vi "GetText.vi"(8 "error in":errorcluster, 11 "Submodule EOL":refnum<class "Submodule EOL.lvclass">) -> (0 "error out":errorcluster, 1 "additional text":string, 2 "text":string, 3 "Submodule EOL out":refnum<class "Submodule EOL.lvclass">, 4 "glyph":string)   [LabVIEW 2025, in "Submodule EOL.lvlib" / "Submodule EOL.lvclass"]
doc: "Returns the text representation of the node used for the tree control.Copyright 2017 National Instruments Corporation\n\nLicensed under the Apache License, Version 2.0 (the \"License\"); you may not use this file except in compliance with the License. You may obtain a copy of the License at http://www.apache.org/licenses/LICENSE-2.0\nUnless required by applicable law or agreed to in writing, software distributed under the License is distributed on an \"AS IS\" BASIS, WITHOUT WARRANTIES OR CONDITIONS OF ANY KIND, either express or implied. See the License for the specific language governing permissions and limitations under the License."
uses:
  Submodule EOL.lvclass
  Submodule EOL.lvclass/Submodule EOL.ctl
  Submodule EOL configuration/Submodule EOL configuration.lvclass/Submodule EOL configuration.ctl
  Submodule EOL configuration/Read Submodule EOL.vi
  Submodule EOL configuration/Submodule EOL configuration.lvclass
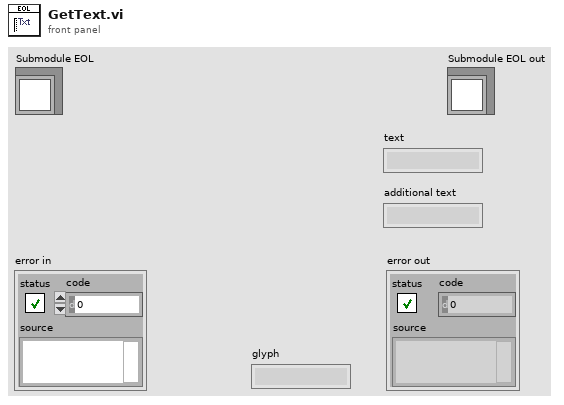
[diagram p1: front panel]
types:
  T1 = typedef "Submodule EOL.lvlib/Submodule EOL configuration.lvclass/Submodule EOL.ctl" = cluster{"PLC Folder Names":string[][], "Timeout Connect OPC":dbl, "Connect OPC Trial":u32, "PLC URL":string, "Digitial IO":string, "HiPOT":string, "ACIR with Switch":string, "DMM with Switch":string, "Ignition Folder Names":string[][], "Ignition URL":string, "Test Name":string}
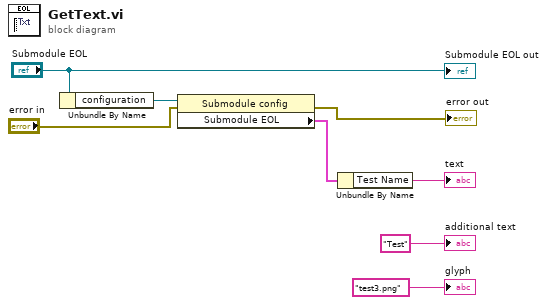
[diagram p0: block diagram]
diagram:
  n1 = Unbundle By Name("Submodule EOL") -> ("configuration"=w5:refnum<class "Submodule EOL configuration.lvclass">)
  n2 = property class="Submodule config"(reference=w5, error in="error in") -> (error out=→"error out":errorcluster, "Submodule EOL"=w4:T1)  [unwired: 1 out]
  n3 = Unbundle By Name(w4) -> ("Test Name"=→"text":string)
  "additional text" <- "Test" ("additional text")
  "glyph" <- "test3.png" ("glyph")
  "Submodule EOL out" <- "Submodule EOL"
